vi "Setpoints.vi"() -> ()   [LabVIEW 2014]
uses:
  <vilib>/Utility/file.llb/Read From Spreadsheet File (DBL).vi
panel:
  out "arm position offset":dbl
  out "wrist position offset":dbl
  in  "Default File":i32
  out "Number of Setpoint Files":i64
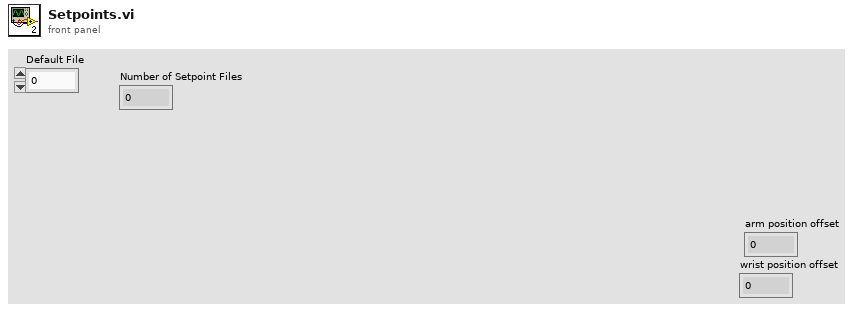
[diagram p1: front panel]
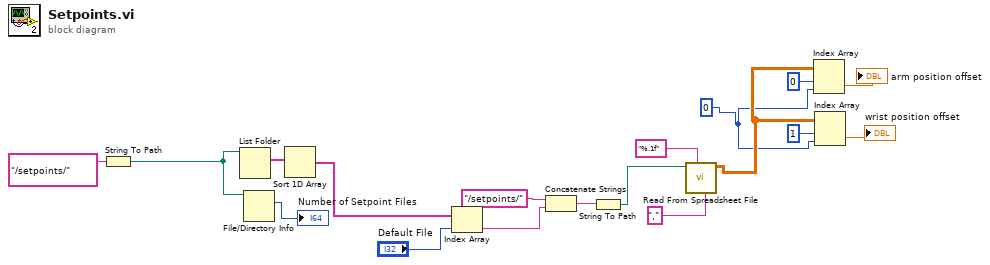
[diagram p0: block diagram]
diagram:
  w1 = 0 ("index (col)")
  n1 = String To Path(string="/setpoints/") -> (path=w10:path)
  n2 = List Folder(path=w10) -> (filenames=w11:string[])  [unwired: 1 in, 5 out]
  n3 = File/Directory Info(path=w10) -> (size=→"Number of Setpoint Files":i64)  [unwired: 1 in, 6 out]
  n4 = Sort 1D Array(array=w11) -> (sorted array=w13:string[])
  n5 = Index Array(array=w13, index="Default File") -> (element=w8:string)
  n6 = Concatenate Strings("/setpoints/" ("string"), w8) -> (w16:string)
  n7 = String To Path(string=w16) -> (path=w15:path)
  n8 = call-poly <vilib>:"Read From Spreadsheet File.vi"("delimiter (\\t)"="," ("delimiter (\\t)"), "format (%.3f)"="%.1f", "file path (dialog if empty)"=w15) -> ("all rows"=w2:dbl[][])  [unwired: 2 in, 6 out]
  n9 = Index Array(array=w2, index (row)=0, index (col)=w1) -> (element=→"arm position offset":dbl)
  n10 = Index Array(array=w2, index (row)=1, index (col)=w1) -> (element=→"wrist position offset":dbl)
